vi "XNET CAN Signal Logger.vi"() -> ()   [LabVIEW 2021]
uses:
  <vilib>/xnet/xnet.llb/XNET Create Session (Signal Input Waveform).vi
  <vilib>/xnet/xnet.llb/XNET Read (Signal Waveform) .vi
  <resource>/objmgr/xnet.rc
panel:
  out "stopped":bool
  out "data":waveform(dbl)[](array[waveform])
  out "Signal Units":string[](array[string])
  out "Signal Values":dbl[](array[numeric])
  in  "Signals to Monitor":string[](array[combo])
  out "#Signals":i32
  in  "Start":bool
  out "error out":errorcluster
  out "Parsed Log file name":string
  in  "Log file name":string="LogFile_{Year}-{Month}-{Day}-{Hour}-{Minute}-{Second}.tdms"
  in  "Log file folder":path=path "C:/Users/NI/Desktop/Data"
  in  "Sample Rate (Hz)":dbl=100.0 format="%#_13g"
  in  "CAN Interface":refnum<k21>="CAN1"
  in  "XNET Cluster":refnum<k21>="ManyXnetChannels"
  in  "stop":bool
  # "Configuration"
  # "Signals to Monitor"
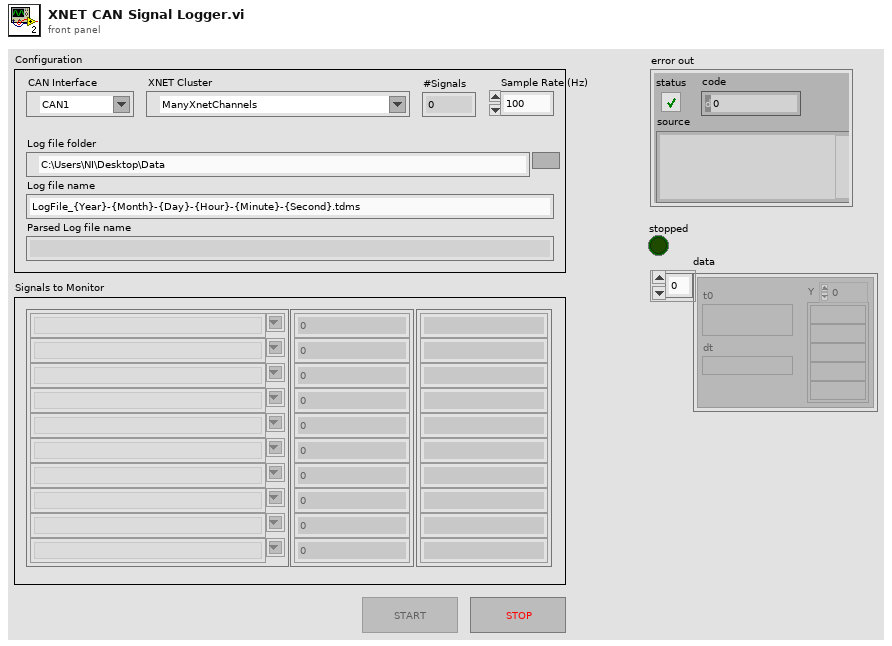
[diagram p1: front panel]
types:
  T1 = enum8{"Enabled", "Disabled", "Disabled and Grayed Out"}
  T2 = enum16{"open", "open or create", "create or replace", "create", "open (read-only)"}
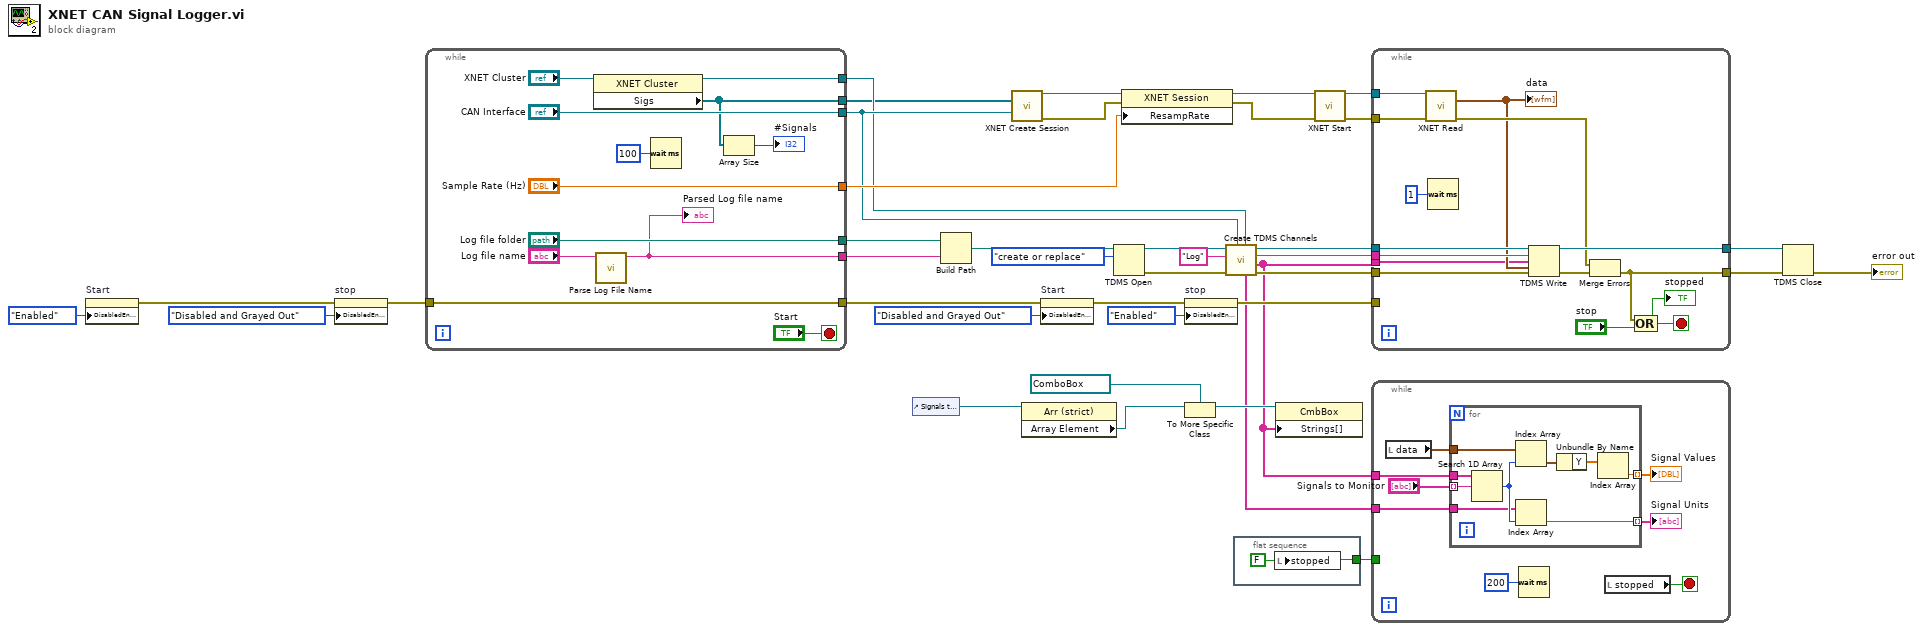
[diagram p0: block diagram]
diagram:
  n1 = property on="Start" class="Bool"("DisabledEnum"=T1."Enabled" ("Disabled")) -> (error out=w9:errorcluster)  [unwired: 2 in, 1 out]
  n2 = property on="stop" class="Bool"(error in=w9, "DisabledEnum"=T1."Disabled and Grayed Out" ("Disabled")) -> (error out=w16:errorcluster)  [unwired: 1 in, 1 out]
  n3 = while {
    tunnel: ["Sample Rate (Hz)"] -> w37
    tunnel: ["Log file folder"] -> w25
    tunnel: [w48] -> w23
    tunnel: ["CAN Interface"] -> w19
    tunnel: [w42] -> w18
    tunnel: w16 -> [w44]
    tunnel: [w44] -> w12
    tunnel: [w40] -> w8
    stop <- "Start" stop-if-true
    n4 = property class="XNET Cluster"(reference="XNET Cluster") -> (reference out=w42:refnum<k21>, "Sigs"=w40:refnum<k21>[])  [unwired: 1 in, 1 out]
    n5 = call "Parse Log File Name.vi"("Log file name"="Log file name") -> ("Parsed Log file name"=w48:string)  [unwired: 10 in]
    "Parsed Log file name" <- w48
    n6 = Wait (ms)(milliseconds to wait=u32 100) -> ()  [unwired: 1 out]
    n7 = Array Size(array=w40) -> (size(s)=→"#Signals":i32)
  }
  n8 = control-ref of="Signals to Monitor"() -> (w7:refnum<vi>)
  n9 = Build Path(base path=w25, name or relative path=w23) -> (appended path=w26:path)
  n10 = call-poly <vilib>:"XNET Create Session.vi"("signal list"=w8, "interface"=w19) -> ("session out"=w39:refnum<k21>, "error out"=w38:errorcluster)  [unwired: 12 in]
  n11 = property class="Arr (strict)"(reference=w7) -> ("Array Element"=w3:refnum<vi>)  [unwired: 1 in, 2 out]
  n12 = property on="Start" class="Bool"(error in=w12, "DisabledEnum"=T1."Disabled and Grayed Out" ("Disabled")) -> (error out=w11:errorcluster)  [unwired: 1 in, 1 out]
  n13 = TDMS Open(10:T2."create or replace" ("operation (0:open)"), 11:w26) -> (0:w29:errorcluster, 3:w31:refnum<k34>)  [unwired: 5 in]
  n14 = property class="XNET Session"(reference=w39, error in=w38, "ResampRate"=w37) -> (reference out=w36:refnum<k21>, error out=w35:errorcluster)
  n15 = property on="stop" class="Bool"(error in=w11, "DisabledEnum"=T1."Enabled" ("Disabled")) -> (error out=w14:errorcluster)  [unwired: 1 in, 1 out]
  n16 = To More Specific Class(target class=refnum<vi> refnum ("Combo Box"), reference=w3) -> (specific class reference=w5:refnum<vi>)  [unwired: 1 in, 1 out]
  n17 = call "Create TDMS Channels.vi"("XNET Cluster"=w18, "CAN Interface"=w19, "error in (no error)"=w29, "group name in"="Log", "TDMS ref in"=w31) -> ("error out"=w28:errorcluster, "Signal Names"=w4:string[], "group name out"=w24:string, "TDMS ref out"=w30:refnum<k34>, "Signal Units"=w2:string[])  [unwired: 2 in]
  n18 = flat-sequence {
    tunnel: [w52] -> w1
    frame #0 {
      w52 = FALSE ("stopped")
      n19 = local write "stopped"(w52) -> ()
    }
  }
  n20 = property class="CmbBox"(reference=w5, "Strings[]"=w4) -> ()  [unwired: 1 in, 2 out]
  n21 = call <vilib>:"XNET Start.vi"("session in"=w36, "error in (no error)"=w35) -> ("session out"=w33:refnum<k21>, "error out"=w34:errorcluster)  [unwired: 12 in]
  n22 = while {
    tunnel: w33 -> [w66]
    tunnel: w34 -> [w65]
    tunnel: [w61] -> w32
    tunnel: w4 -> [w53]
    tunnel: w30 -> [w59]
    tunnel: w28 -> [w58]
    tunnel: w24 -> [w57]
    tunnel: [w55] -> w21
    tunnel: w14 -> [_]
    stop <- w63 stop-if-true
    n23 = call-poly <vilib>:"XNET Read.vi"("session in"=w66, "error in (no error)"=w65) -> ("data"=w54:waveform(dbl)[], "error out"=w56:errorcluster)  [unwired: 11 in, 1 out]
    "data" <- w54
    n24 = Wait (ms)(milliseconds to wait=u32 1) -> ()  [unwired: 1 out]
    n25 = TDMS Write(0:w59, 5:w57, 7:w53, 9:w54, 11:w58) -> (4:w61:refnum<k34>, 15:w60:errorcluster)  [unwired: 1 in, 2 out]
    n26 = Merge Errors(w56, w60) -> (w55:errorcluster)
    n27 = Compound Arithmetic op=OR(w55, "stop") -> (w63:bool)
    "stopped" <- w63
  }
  n28 = while {
    tunnel: w4 -> [w74]
    tunnel: w2 -> [w70]
    tunnel: w1 -> [_]
    stop <- w67 stop-if-true
    n29 = local read "data"() -> (w69:waveform(dbl)[])
    n30 = for {
      tunnel: "Signals to Monitor" -> [w83] mode=indexing
      tunnel: w74 -> [w82]
      tunnel: w69 -> [w81]
      tunnel: [w79] -> w72 mode=indexing
      tunnel: w70 -> [w76]
      tunnel: [w75] -> w73 mode=indexing
      n31 = Search 1D Array(1D array=w82, element=w83) -> (index of element=w77:i32)  [unwired: 1 in]
      n32 = Index Array(array=w81, index=w77) -> (element=w78:waveform(dbl))
      n33 = Index Array(array=w76, index=w77) -> (element=w75:string)
      n34 = Unbundle By Name(w78) -> ("Y"=w80:dbl[])
      n35 = Index Array(array=w80) -> (element=w79:dbl)  [unwired: 1 in]
    }
    "Signal Values" <- w72
    "Signal Units" <- w73
    n36 = Wait (ms)(milliseconds to wait=u32 200) -> ()  [unwired: 1 out]
    n37 = local read "stopped"() -> (w67:bool)
  }
  n38 = TDMS Close(8:w21, 11:w32) -> (0:→"error out":errorcluster)  [unwired: 1 out]
